vi "Init.vi"(0 "reference in":refnum<class "FPGA_Concrete.lvclass">, 11 "error in (no error)":errorcluster) -> (4 "reference out":refnum<class "FPGA_Concrete.lvclass">, 15 "error out":errorcluster)   [LabVIEW 2019, in "FPGA_Concrete.lvclass"]
uses:
  FPGA_Concrete.lvclass
  FPGA VI Reference.ctl
  FPGA_Concrete.lvclass/FPGA_Concrete.ctl
  <vilib>/FPGAPlugInAG/cRIO-9035/niLvFpga_Open_cRIO-9035.vi
  <vilib>/rvi/interface/common/dynamic/niFpgaDynamicAddResources.vi
  <vilib>/rvi/interface/common/niFpgaWaitOnOcc.vi
  <vilib>/Utility/error.llb/Error Cluster From Error Code.vi
  <vilib>/rvi/interface/nirviOpenFPGA/nirviOpenFPGA.xnode
  FPGA Bitfiles/hydrort_FPGATarget_MAINFPGA_+-Tm9L0us+s.lvbitx
  <vilib>/rvi/interface/nirviMethod/nirviMethod.xnode
  <vilib>/rvi/errors/niLvFpgaMergeErrorWithErrorCode.vi
  <vilib>/FPGAPlugInAG/Dynamic/niLvFpga_ConfigureFifo_Dynamic.vi
  <vilib>/FPGAPlugInAG/Dynamic/niLvFpga_StartFifo_Dynamic.vi
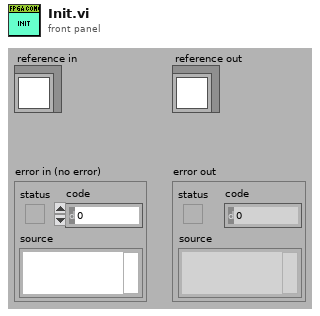
[diagram p1: front panel]
types:
  T1 = typedef "FPGA_Concrete.lvclass/FPGA VI Reference.ctl" = refnum<k20>
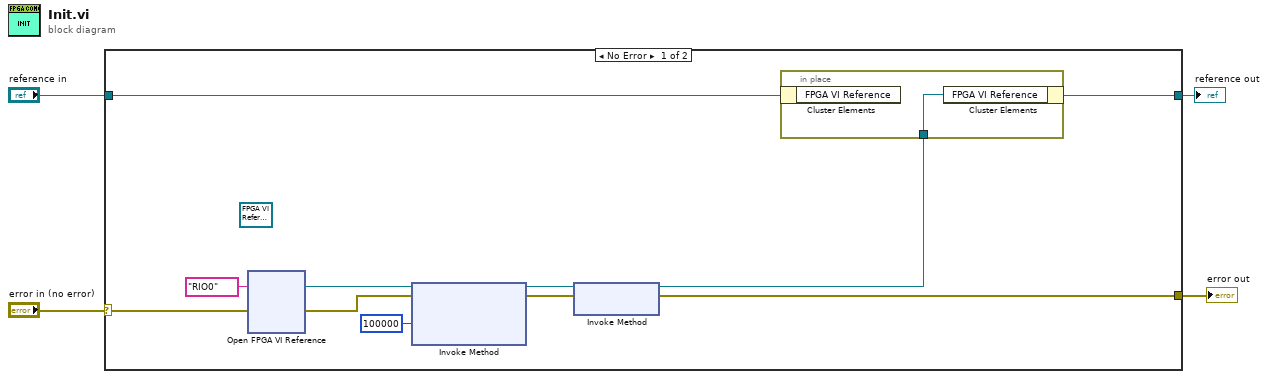
[diagram p0: block diagram]
diagram:
  n1 = case shown="No Error" "error in (no error)" {
    selector: "error in (no error)" -> [w15 w18]
    tunnel: [w5 w18] -> w3
    tunnel: [w13 w17] -> w1
    tunnel: "reference in" -> [w14 w17]
    frame No Error {
      (unwired) T1 refnum ("FPGA VI Reference")
      n2 = xnode "Open FPGA VI Reference"("error in"=w15, "resource name"=tag "RIO0") -> ("FPGA VI Reference Out"=w11:refnum<k20>, "error out"=w10:errorcluster)
      n3 = xnode "Invoke Method"("FPGA VI Reference In"=w11, "error in"=w10, "Requested Depth"=u32 100000) -> ("FPGA VI Reference Out"=w8:refnum<k20>, "error out"=w7:errorcluster)  [unwired: 1 out]
      n4 = xnode "Invoke Method"("FPGA VI Reference In"=w8, "error in"=w7) -> ("FPGA VI Reference Out"=w6:refnum<k20>, "error out"=w5:errorcluster)
      n5 = in-place {
        in-place-border: w6 -> [w16]
        n6 = in-place-cluster #1(w14) -> ()  [unwired: 1 out]
        n7 = in-place-cluster #1("FPGA VI Reference"=w16) -> (w13:refnum<class "FPGA_Concrete.lvclass">)
      }
    }
    frame Error {
    }
  }
  "error out" <- w3
  "reference out" <- w1
